vi "Init AI.vi"(7 "DAQmx Physical Channel":tag, 8 "error in (no error)":errorcluster, 9 "label":string="tmp", 10 "task in":refnum<k21>, 11 "DAQmx Scale Name":tag) -> (0 "error out":errorcluster, 3 "Task Out":refnum<k21>)   [LabVIEW 2015]
uses:
  <vilib>/DAQmx/create/channels.llb/DAQmx Create Channel (AI-Voltage-Basic).vi
  <resource>/objmgr/daqmx.rc
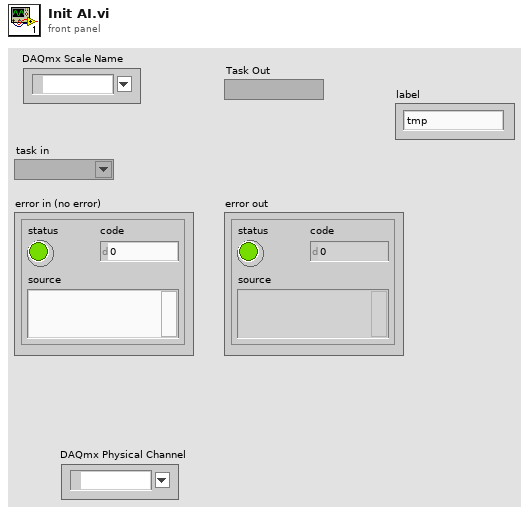
[diagram p1: front panel]
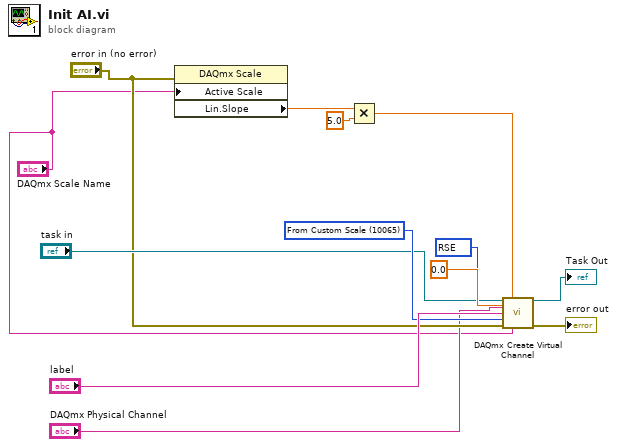
[diagram p0: block diagram]
diagram:
  w8 = 10065 items=["Volts"=10348, "From Custom Scale"=10065] ("units")
  w7 = 10083 items=["Default"=-1, "RSE"=10083, "NRSE"=10078, "Differential"=10106, "Pseudodifferential"=12529] ("input terminal configuration")
  n1 = property class="DAQmx Scale"(error in="error in (no error)", "Active Scale"="DAQmx Scale Name") -> ("Lin.Slope"=w10:dbl)  [unwired: 1 in, 2 out]
  n2 = Multiply(x=w10, y=5.0) -> (x*y=w12:dbl)
  n3 = call-poly <vilib>:"DAQmx Create Virtual Channel.vi"("task in"="task in", "maximum value"=w12, "minimum value"=0.0, "input terminal configuration"=w7, "physical channels"="DAQmx Physical Channel", "name to assign"="label", "units"=w8, "error in"="error in (no error)", "custom scale name"="DAQmx Scale Name") -> ("task out"=→"Task Out":refnum<k21>, "error out"=→"error out":errorcluster)  [unwired: 5 in]
